vi "Configure Runt Trigger Source [RT] Core.vi"(0 "IVI_Scope in":refnum<class "IVI_Scope.lvclass">, 5 "trigger source (\"CHANNEL1\")":string(combo)="CHANNEL1", 7 "runt low threshold (1.0 V)":dbl[unit]=1.0 format="%.3f", 9 "runt high threshold (4.0 V)":dbl[unit]=4.0 format="%.3f", 11 "error in (no error)":errorcluster) -> (4 "IVI_Scope out":refnum<class "IVI_Scope.lvclass">, 15 "error out":errorcluster)   [LabVIEW 2015, in "IVI_Scope.lvlib" / "IVI_Scope.lvclass"]
doc: "This VI configures the runt trigger. A runt trigger occurs when the trigger signal you specify with the Runt Trigger Source parameter crosses one of the runt thresholds twice without crossing the other runt threshold. You specify the runt thresholds with the Runt Low Threshold and Runt High Threshold parameters. You specify the polarity of the runt with the Runt Polarity parameter.\n\nNote \n(1) This VI affects instrument behavior only if the trigger type is\n IVISCOPE_VAL_RUNT_TRIGGER. Call the IviScope Configure Trigger\n and IviScope Configure Trigger Coupling VIs to set the trigger type and\n trigger coupling before calling this VI.\n\n(2) This VI is part of the IviScopeRuntTrigger [RT] extension group."
uses:
  IVI_Scope.lvclass
  IVI_Scope.lvclass/IVI_Scope.ctl
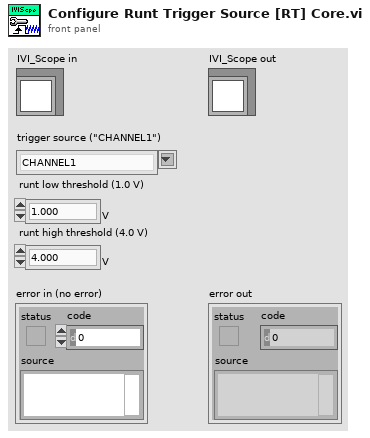
[diagram p1: front panel]
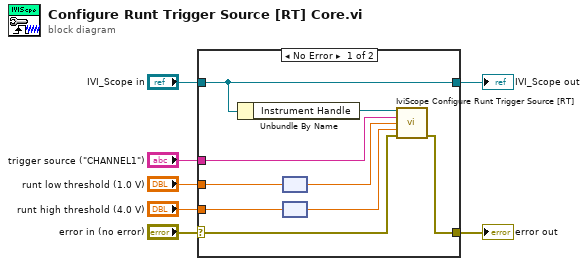
[diagram p0: block diagram]
diagram:
  n1 = case shown="No Error" "error in (no error)" {
    selector: "error in (no error)" -> [w14 w18]
    tunnel: [w13 w18] -> w6
    tunnel: [w16 w17] -> w4
    tunnel: "IVI_Scope in" -> [w16 w17]
    tunnel: "trigger source (\"CHANNEL1\")" -> [w12 _]
    tunnel: "runt low threshold (1.0 V)" -> [w11 _]
    tunnel: "runt high threshold (4.0 V)" -> [w10 _]
    frame No Error {
      n2 = Unbundle By Name(w16) -> ("Instrument Handle"=w15:refnum<k15>)
      n3 = node(w11) -> (w9:dbl)
      n4 = node(w10) -> (w8:dbl)
      n5 = call <vilib>:"IviScope Configure Runt Trigger Source [RT].vi"("instrument handle"=w15, "trigger source (\"CHANNEL1\")"=w12, "runt low threshold (1.0 V)"=w9, "runt high threshold (4.0 V)"=w8, "error in (no error)"=w14) -> ("error out"=w13:errorcluster)  [unwired: 9 in, 1 out]
    }
    frame Error {
    }
  }
  "error out" <- w6
  "IVI_Scope out" <- w4
